vi "appendXMLTarget.vi"(8 "Target":cluster{"X Target":sgl, "Y Target":sgl}, 9 "error in (no error)":errorcluster, 10 "Parent Camera Node":refnum<k20>, 11 "DOM document in":refnum<k20>) -> (0 "error out":errorcluster)   [LabVIEW 2013]
uses:
  <resource>/objmgr/DOMUserDefRef.rc
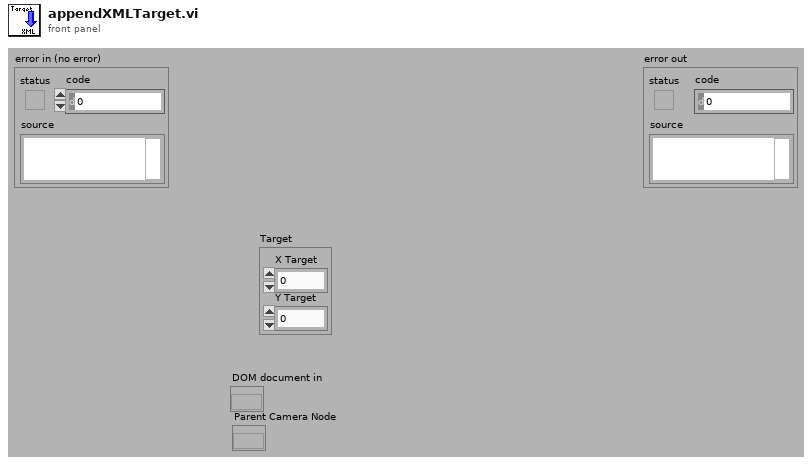
[diagram p1: front panel]
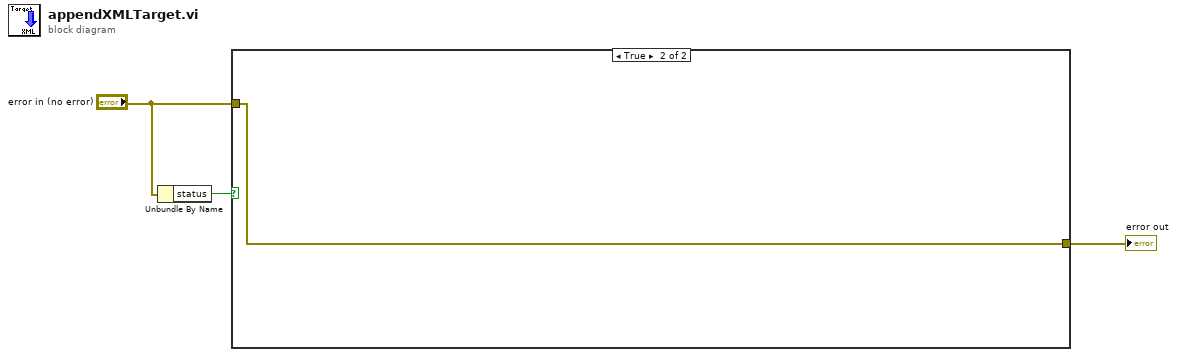
[diagram p0: block diagram]
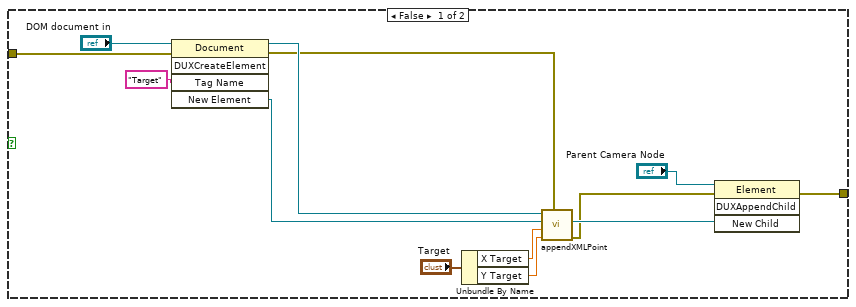
[diagram p2: hidden frame]
diagram:
  n1 = Unbundle By Name("error in (no error)") -> ("status"=w2:bool)
  n2 = case shown="True" w2 {
    tunnel: "error in (no error)" -> [w5 w17]
    tunnel: [w4 w17] -> w3
    frame False {
      n3 = invoke class="Document" method="DUXCreateElement"(reference="DOM document in", error in=w5, "Tag Name"="Target") -> (reference out=w8:refnum<k20>, error out=w6:errorcluster, "New Element"=w11:refnum<k20>)  [unwired: 2 in, 2 out]
      n4 = Unbundle By Name("Target") -> ("X Target"=w15:sgl, "Y Target"=w14:sgl)
      n5 = call "appendXMLPoint.vi"("error in (no error)"=w6, "y"=w14, "x"=w15, "Parent Node"=w11, "DOM document in"=w8) -> ("error out"=w7:errorcluster, "Parent Node Out"=w9:refnum<k20>)  [unwired: 4 in]
      n6 = invoke class="Element" method="DUXAppendChild"(reference="Parent Camera Node", error in=w7, "New Child"=w9) -> (error out=w4:errorcluster)  [unwired: 1 in, 3 out]
    }
    frame True {
    }
  }
  "error out" <- w3
